vi "Introspection Output.vi"(8 "error in (no error)":errorcluster, 11 "ONNX Class in":refnum<class "ONNX Class.lvclass">) -> (0 "error out":errorcluster, 2 "Introspection Output":T1, 3 "ONNX Class out":refnum<class "ONNX Class.lvclass">)   [LabVIEW 2017, in "ONNX Class Library.lvlib" / "ONNX Class.lvclass"]
uses:
  ONNX Class.lvclass
  ONNX Class.lvclass/ONNX Class.ctl
  ONNX Class Library.lvlib
  TypeDef/IO.ctl
  TypeDef/Introspection.ctl
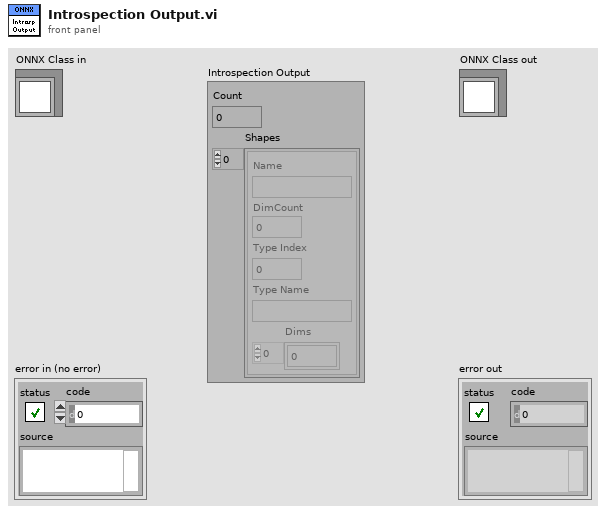
[diagram p1: front panel]
types:
  T1 = typedef "ONNX Class Library.lvlib/Introspection.ctl" = cluster{"Count":i32, "Shapes":T2[]}
  T2 = typedef "ONNX Class Library.lvlib/IO.ctl" = cluster{"Name":string, "DimCount":i32, "Type Index":i32, "Type Name":string, "Dims":i64[]}
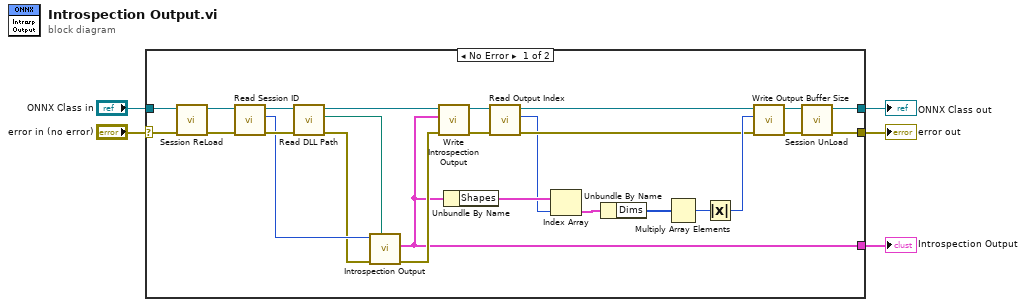
[diagram p0: block diagram]
diagram:
  n1 = case shown="No Error" "error in (no error)" {
    selector: "error in (no error)" -> [w29 w33]
    tunnel: [w19 w33] -> w4
    tunnel: [w20 w32] -> w2
    tunnel: "ONNX Class in" -> [w30 w32]
    tunnel: [w12 _] -> w1
    frame No Error {
      n2 = call-dynamic "Session ReLoad.vi"("error in (no error)"=w29, "ONNX Class in"=w30) -> ("error out"=w27:errorcluster, "ONNX Class out"=w28:refnum<class "ONNX Class.lvclass">)  [unwired: 8 in]
      n3 = call-dynamic "Read Session ID.vi"("error in (no error)"=w27, "ONNX Class in"=w28) -> ("error out"=w25:errorcluster, "Session ID"=w24:i32, "ONNX Class out"=w26:refnum<class "ONNX Class.lvclass">)  [unwired: 7 in]
      n4 = call-dynamic "Read DLL Path.vi"("error in (no error)"=w25, "ONNX Class in"=w26) -> ("error out"=w23:errorcluster, "DLL Path"=w22:path, "ONNX Class out"=w21:refnum<class "ONNX Class.lvclass">)  [unwired: 7 in]
      n5 = call "Introspection Output.vi"("DLL path"=w22, "error in (no error)"=w23, "session id in"=w24) -> ("error out"=w31:errorcluster, "Introspection Output"=w12:T1)  [unwired: 6 in, 1 out]
      n6 = call-dynamic "Write Introspection Output.vi"("error in (no error)"=w31, "Introspection"=w12, "ONNX Class in"=w21) -> ("error out"=w9:errorcluster, "ONNX Class out"=w10:refnum<class "ONNX Class.lvclass">)  [unwired: 7 in]
      n7 = Unbundle By Name(w12) -> ("Shapes"=w18:T2[])
      n8 = call-dynamic "Read Output Index.vi"("error in (no error)"=w9, "ONNX Class in"=w10) -> ("error out"=w7:errorcluster, "Output Index"=w6:i32, "ONNX Class out"=w8:refnum<class "ONNX Class.lvclass">)  [unwired: 7 in]
      n9 = Index Array(array=w18, index=w6) -> (element=w17:T2)
      n10 = Unbundle By Name(w17) -> ("Dims"=w16:i64[])
      n11 = Multiply Array Elements(1:w16) -> (0:w15:i64)
      n12 = Absolute Value(x=w15) -> (abs(x)=w11:i64)
      n13 = call-dynamic "Write Output Buffer Size.vi"("error in (no error)"=w7, "Output Buffer Size"=w11, "ONNX Class in"=w8) -> ("error out"=w13:errorcluster, "ONNX Class out"=w14:refnum<class "ONNX Class.lvclass">)  [unwired: 7 in]
      n14 = call-dynamic "Session UnLoad.vi"("error in (no error)"=w13, "ONNX Class in"=w14) -> ("error out"=w19:errorcluster, "ONNX Class out"=w20:refnum<class "ONNX Class.lvclass">)  [unwired: 8 in]
    }
    frame Error {
    }
  }
  "error out" <- w4
  "ONNX Class out" <- w2
  "Introspection Output" <- w1
